vi "Transport.vi"(4 "Queue of Error":refnum<queue>, 6 "Queue of Self Attributes":refnum<queue>, 7 "Actor in":refnum<class "Actor.lvclass">, 10 "Attributes":refnum<class "Attributes.lvclass">) -> (0 "Error out":errorcluster, 5 "Actor out":refnum<class "Actor.lvclass">)   [LabVIEW 2025, in "jettl.lvlib" / "Transport.lvlib" / "Notifier.lvlib"]
uses:
  Notifier.lvlib
  jettl.lvlib
  Actor/Actor.lvclass
  Attributes/Attributes/Attributes.lvclass
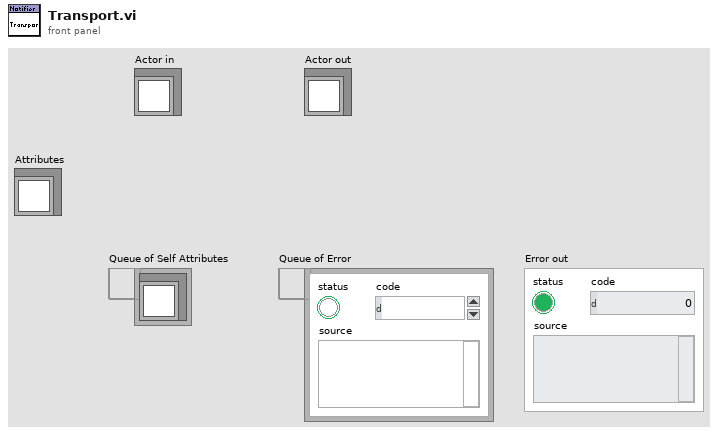
[diagram p1: front panel]
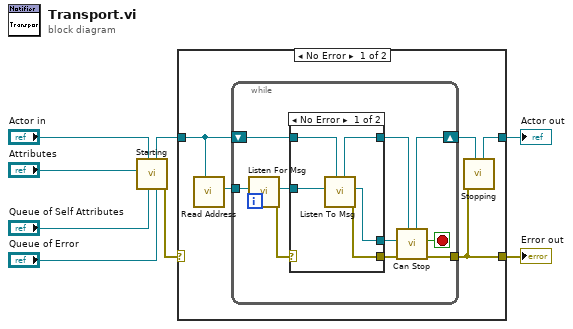
[diagram p0: block diagram]
diagram:
  n1 = call "Starting.vi"("Queue of Error"="Queue of Error", "Queue of Self Attributes"="Queue of Self Attributes", "Actor in"="Actor in", "Attributes"="Attributes") -> ("Error out"=w4:errorcluster, "Actor out"=w5:refnum<class "Actor.lvclass">)  [unwired: 6 in]
  n2 = case shown="No Error" w4 {
    selector: w4 -> [_ w31]
    tunnel: [w11 w32] -> w7
    tunnel: w5 -> [w10 w32]
    tunnel: [w13 w31] -> w8
    frame No Error {
      n3 = call "Read Address.vi"("Actor"=w10) -> ("Address"=w9:refnum<data-value>)  [unwired: 10 in]
      n4 = while {
        shift-right: [w21] -> w12
        shift-left: w10 -> [w19]
        tunnel: [w22] -> w13
        tunnel: w9 -> [w17]
        stop <- w20 stop-if-true
        n5 = call "Listen For Msg.vi"("Address"=w17) -> ("Error out"=w16:errorcluster, "Msg"=w15:refnum<class "Msg.lvclass">)  [unwired: 9 in]
        n6 = case shown="No Error" w16 {
          selector: w16 -> [_ w29]
          tunnel: [w25 w29] -> w23
          tunnel: w19 -> [w28 w30]
          tunnel: [w26 w30] -> w18
          tunnel: w15 -> [w27 _]
          tunnel: [w24 _] -> w14
          frame No Error {
            n7 = call "Listen To Msg.vi"("Actor in"=w28, "Msg"=w27) -> ("Error out"=w25:errorcluster, "Msg Output"=w24:refnum<class "Msg Output.lvclass">, "Actor out"=w26:refnum<class "Actor.lvclass">)  [unwired: 7 in]
          }
          frame Error {
          }
        }
        n8 = call "Can Stop.vi"("Actor in"=w18, "Error in"=w23, "Msg Output"=w14) -> ("Error out"=w22:errorcluster, "Stop"=w20:bool, "Actor out"=w21:refnum<class "Actor.lvclass">)  [unwired: 6 in]
      }
      n9 = call "Stopping.vi"("Actor in"=w12, "Error in"=w13) -> ("Actor out"=w11:refnum<class "Actor.lvclass">)  [unwired: 9 in]
    }
    frame Error {
    }
  }
  "Error out" <- w8
  "Actor out" <- w7
